vi "Manipulate Active Pixels.vi"(6 "Advance Line":bool, 7 "Rotate":bool, 8 "error in (no error)":errorcluster, 9 "Right":bool, 10 "Left":bool, 11 "Game Engine in":refnum<class "Game Engine.lvclass">) -> (0 "error out":errorcluster, 3 "Game Engine out":refnum<class "Game Engine.lvclass">)   [LabVIEW 2017, in "Game Engine.lvlib" / "Game Engine.lvclass"]
uses:
  Game Engine.lvclass
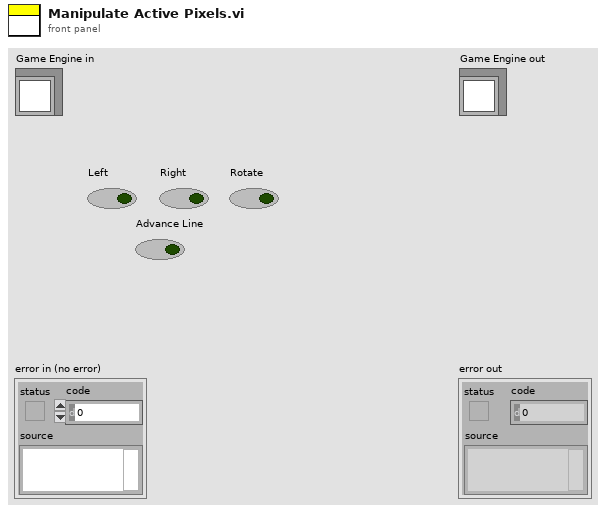
[diagram p1: front panel]
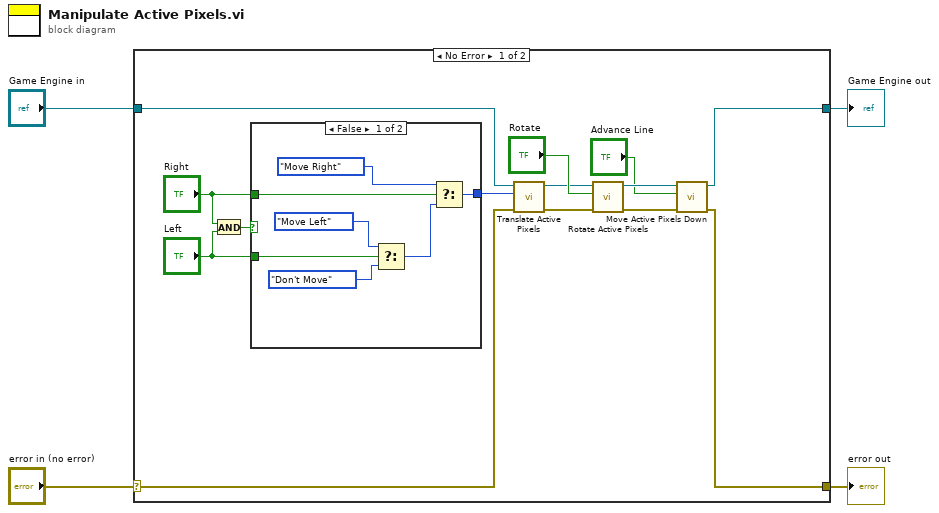
[diagram p0: block diagram]
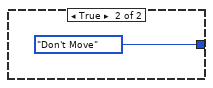
[diagram p2: hidden frame]
diagram:
  n1 = case shown="No Error" "error in (no error)" {
    selector: "error in (no error)" -> [w8 w28]
    tunnel: [w5 w28] -> w3
    tunnel: [w11 w27] -> w1
    tunnel: "Game Engine in" -> [w10 w27]
    frame No Error {
      n2 = And(x="Right", y="Left") -> (x .and. y?=w18:bool)
      n3 = case shown="False" w18 {
        tunnel: "Right" -> [w24 _]
        tunnel: "Left" -> [w22 _]
        tunnel: [w19 enum16{"Move Left", "Don't Move", "Move Right"}."Don't Move"] -> w9
        frame False {
          n4 = Select(t=enum16{"Move Left", "Don't Move", "Move Right"}."Move Left", s=w22, f=enum16{"Move Left", "Don't Move", "Move Right"}."Don't Move") -> (s? t:f=w21:enum16{"Move Left", "Don't Move", "Move Right"})
          n5 = Select(t=enum16{"Move Left", "Don't Move", "Move Right"}."Move Right", s=w24, f=w21) -> (s? t:f=w19:enum16{"Move Left", "Don't Move", "Move Right"})
        }
        frame True {
        }
      }
      n6 = call "Translate Active Pixels.vi"("error in (no error)"=w8, "Enum"=w9, "Game Engine in"=w10) -> ("error out"=w7:errorcluster, "Game Engine out"=w6:refnum<class "Game Engine.lvclass">)  [unwired: 7 in]
      n7 = call "Rotate Active Pixels.vi"("error in (no error)"=w7, "Rotate"="Rotate", "Game Engine in"=w6) -> ("error out"=w13:errorcluster, "Game Engine out"=w14:refnum<class "Game Engine.lvclass">)  [unwired: 7 in]
      n8 = call "Move Active Pixels Down.vi"("error in (no error)"=w13, "Boolean"="Advance Line", "Game Engine in"=w14) -> ("error out"=w5:errorcluster, "Game Engine out"=w11:refnum<class "Game Engine.lvclass">)  [unwired: 7 in]
    }
    frame Error {
    }
  }
  "error out" <- w3
  "Game Engine out" <- w1
